vi "AirFlow.vi"(0 "Stack Height (m)":dbl, 1 "Louver Position (% Open)":dbl, 2 "Time Interval (s)":dbl, 3 "NDHX Tube Pitch (m)":dbl, 4 "Air Cold Temperature (K)":dbl, 5 "NDHX Tube Diameter (m)":dbl, 6 "NDHX Tube Length (m)":dbl, 7 "Stack Inner Diameter (m)":dbl, 8 "Air Hot Temperature (K)":dbl, 9 "NDHX Number of Tubes":dbl, 11 "Air Mass Flow (kg/s)":dbl, 12 "NDHX Heat Transfer (W)":dbl) -> (10 "Cp of Air (J/kgK)":dbl, 13 "Air Inlet Density (kg/m^3)":dbl, 14 "Air Ave Temperature (C)":dbl, 15 "Air Inlet Viscosity (Pa-s)":dbl, 16 "Air Temperature Delta (K)":dbl, 17 "Air Mass Flow (kg/s)":dbl, 18 "Air Outlet Density (kg/m^3)":dbl, 19 "Air Inlet Velocity (kg/m^3)":dbl, 20 "Air Outlet Viscosity (Pa-s)":dbl, 21 "Heat Rejection (W)":dbl, 22 "Air Outlet Velocity (kg/m^3)":dbl, 23 "Air Outlet Temperature (K)":dbl, 24 "Air Average Viscosity (Pa-s)":dbl, 25 "Air Average Density (kg/m^3)":dbl, 26 "Air Average Velocity (kg/m^3)":dbl)   [LabVIEW 2019]
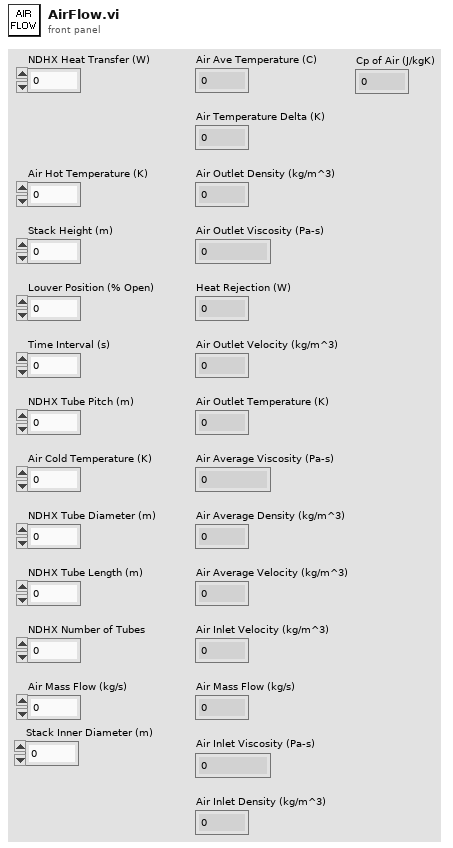
[diagram p1: front panel]
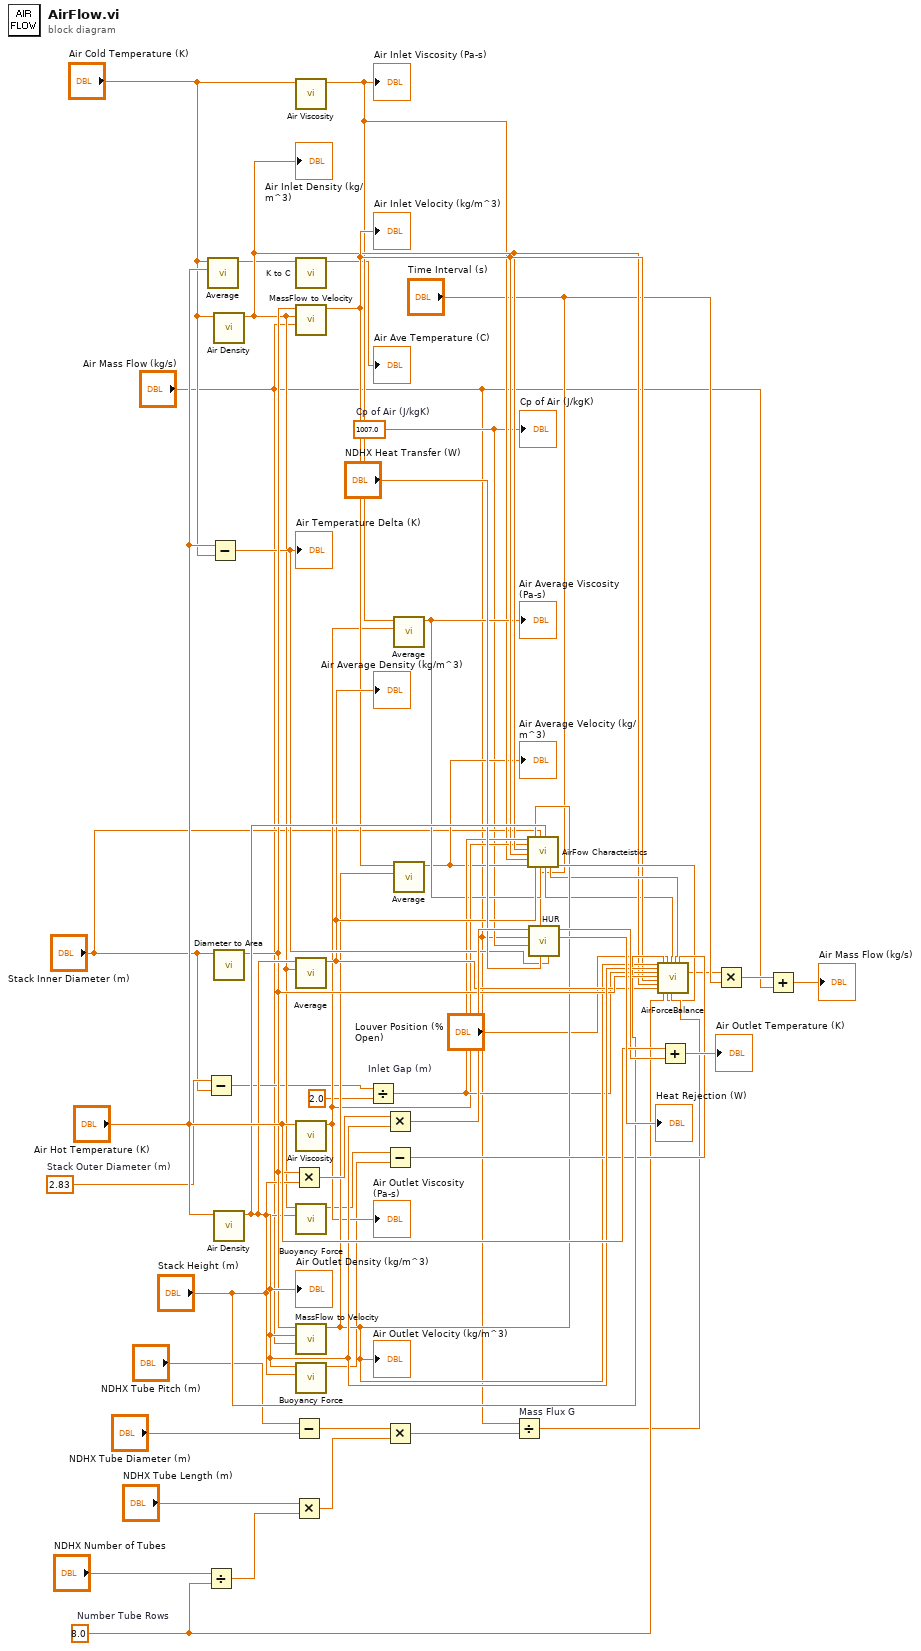
[diagram p0: block diagram]
diagram:
  w6 = 1007.0  # Cp of Air (J/kgK)
  w37 = 8.0  # Number Tube Rows
  w10 = 2.83  # Stack Outer Diameter (m)
  n1 = Subtract(x=w10, y="Stack Inner Diameter (m)") -> (x-y=w14:dbl)
  n2 = Divide(x="NDHX Number of Tubes", y=w37) -> (x/y=w38:dbl)
  n3 = call "Average.vi"("Number 2"="Air Hot Temperature (K)", "Number 1"="Air Cold Temperature (K)") -> ("Average"=w8:dbl)  [unwired: 9 in]
  n4 = Subtract(x="Air Hot Temperature (K)", y="Air Cold Temperature (K)") -> (x-y=w40:dbl)
  "Air Temperature Delta (K)" <- w40
  n5 = call "Air Density.vi"("Temperature (K)"="Air Cold Temperature (K)") -> ("Density (kg/m^3)"=w28:dbl)  [unwired: 10 in]
  "Air Inlet Density (kg/m^3)" <- w28
  n6 = call "Diameter to Area.vi"("Diameter (m)"="Stack Inner Diameter (m)") -> ("Area (m^2)"=w43:dbl)  [unwired: 10 in]
  n7 = call "Air Density.vi"("Temperature (K)"="Air Hot Temperature (K)") -> ("Density (kg/m^3)"=w44:dbl)  [unwired: 10 in]
  "Air Outlet Density (kg/m^3)" <- w44
  n8 = Multiply(x=w43, y="Stack Height (m)") -> (x*y=w45:dbl)
  n9 = Subtract(x="NDHX Tube Pitch (m)", y="NDHX Tube Diameter (m)") -> (x-y=w24:dbl)
  n10 = Multiply(x="NDHX Tube Length (m)", y=w38) -> (x*y=w23:dbl)
  n11 = call "Air Viscosity.vi"("Temperature (K)"="Air Cold Temperature (K)") -> ("Viscosity (Pa-s)"=w17:dbl)  [unwired: 10 in]
  "Air Inlet Viscosity (Pa-s)" <- w17
  n12 = call "K to C.vi"("Temperature (K)"=w8) -> ("Temperature (C)"=→"Air Ave Temperature (C)":dbl)  [unwired: 10 in]
  n13 = call "MassFlow to Velocity.vi"("Mass Flow (kg/s)"="Air Mass Flow (kg/s)", "Density (kg/m^3)"=w28, "Area (m^2)"=w43) -> ("Velocity (m/s)"=w29:dbl)  [unwired: 8 in]
  "Air Inlet Velocity (kg/m^3)" <- w29
  n14 = call "Average.vi"("Number 2"=w28, "Number 1"=w44) -> ("Average"=w35:dbl)  [unwired: 9 in]
  "Air Average Density (kg/m^3)" <- w35
  n15 = call "Air Viscosity.vi"("Temperature (K)"="Air Hot Temperature (K)") -> ("Viscosity (Pa-s)"=w19:dbl)  [unwired: 10 in]
  "Air Outlet Viscosity (Pa-s)" <- w19
  n16 = call "Buoyancy Force.vi"("Height (m)"="Stack Height (m)", "Density (kg/m^3)"=w28) -> ("Potential (Pa)"=w12:dbl)  [unwired: 9 in]
  n17 = call "MassFlow to Velocity.vi"("Mass Flow (kg/s)"="Air Mass Flow (kg/s)", "Density (kg/m^3)"=w44, "Area (m^2)"=w43) -> ("Velocity (m/s)"=w32:dbl)  [unwired: 8 in]
  "Air Outlet Velocity (kg/m^3)" <- w32
  n18 = call "Buoyancy Force.vi"("Height (m)"="Stack Height (m)", "Density (kg/m^3)"=w44) -> ("Potential (Pa)"=w13:dbl)  [unwired: 9 in]
  n19 = Divide "Inlet Gap (m)"(x=w14, y=2.0) -> (x/y=w30:dbl)
  n20 = Multiply(x=w45, y=w44) -> (x*y=w46:dbl)
  n21 = Subtract(x=w12, y=w13) -> (x-y=w39:dbl)
  n22 = Multiply(x=w24, y=w23) -> (x*y=w25:dbl)
  n23 = call "Average.vi"("Number 2"=w19, "Number 1"=w17) -> ("Average"=w18:dbl)  [unwired: 9 in]
  "Air Average Viscosity (Pa-s)" <- w18
  n24 = call "Average.vi"("Number 2"=w32, "Number 1"=w29) -> ("Average"=w16:dbl)  [unwired: 9 in]
  "Air Average Velocity (kg/m^3)" <- w16
  n25 = Divide "Mass Flux G"(x="Air Mass Flow (kg/s)", y=w25) -> (x/y=w34:dbl)
  n26 = call "AirFow Characteistics.vi"("Numeric in"=w30, "Viscosity (Pa-s)"=w19, "Density (kg/m^3) 2"=w28, "Velocity (m/s) 2"=w29, "Viscosity (Pa-s) 2"=w17, "Average 3"=w16, "Velocity (m/s)"=w32, "Average"=w35, "Stack Inner Diameter (m)"="Stack Inner Diameter (m)", "Average 2"=w18, "Density (kg/m^3)"=w44) -> ("Friction Factor 2"=w27:dbl, "Friction Factor"=w31:dbl, "Numeric out"=w33:dbl)  [unwired: 6 out]
  n27 = call "HUR.vi"("Delta T (K)"=w40, "Heating Power (W)"="NDHX Heat Transfer (W)", "Time"="Time Interval (s)", "Cp (J/kgK)"=w6, "Mass Flow (kg/s)"="Air Mass Flow (kg/s)", "Hot Mass (kg)"=w46) -> ("Cooling Power (W)"=→"Heat Rejection (W)":dbl, "HUR (K)"=w48:dbl)  [unwired: 3 in, 1 out]
  n28 = call "AirForceBalance.vi"("Velocity (m/s)"=w32, "Density (kg/m^3)"=w44, "Numeric 5"=w30, "NDHX XSection Area (m^2)"=w43, "Velocity (m/s) 2"=w29, "Density (kg/m^3) 2"=w28, "Average"=w35, "Stack Height (m)"="Stack Height (m)", "Number Tube Rows"=w37, "Louver Position (% Open)"="Louver Position (% Open)", "Numeric 4"=w33, "Friction Factor 2"=w27, "Numeric 3"=w34, "Friction Factor"=w31, "Thermal Driving Force (Pa)"=w39) -> ("Air Mass Acceleration (kg/s^2)"=w4:dbl)  [unwired: 6 in, 6 out]
  n29 = Add(x="Air Hot Temperature (K)", y=w48) -> (x+y=→"Air Outlet Temperature (K)":dbl)
  n30 = Multiply(x=w4, y="Time Interval (s)") -> (x*y=w3:dbl)
  n31 = Add(x=w3, y="Air Mass Flow (kg/s)") -> (x+y=→"Air Mass Flow (kg/s)":dbl)
  "Cp of Air (J/kgK)" <- w6
